vi "Set__slk_mt.vi"(7 "values":string[][](array[string]), 8 "error in (no error)":errorcluster, 11 "ring in":refnum<class "Ring__slk_mt.lvclass">) -> (0 "error out":errorcluster, 3 "ring out":refnum<class "Ring__slk_mt.lvclass">)   [LabVIEW 2013, in "Lazyboots Menu Tool.lvlib" / "Ring__slk_mt.lvclass"]
doc: "Sets the values to the control on GUI.\n\n<b>Values:</b>\n[ [Section, Key, Value], [Section, Key, Value], ..., [Section, Key, Value] ]"
uses:
  Ring__slk_mt.lvclass
  TypeDef/TypeDef_ConnectorPattern__slk_mt.ctl
  Library/Lazyboots Menu Tool.lvlib
panel:
  # "Set__slk_mt.vi\nSets the values to the control on GUI.\n\nNOTICE -- YOU MUST LEAVE THIS NOTICE IN PLACE.\n\nCopyright (c) 2011, LIANG LIU Shawn.Liu.cn@gmail.com\nAll rights reserved.\n\nRedistribution and use in source and binary forms, with or without modification, are permitted provided that the following conditions are met:\n-Redistributions of source code must retain the above copyright notice, this list of conditions and the following disclaimer.\n-Redistributions in binary form must reproduce the above copyright notice, this list of conditions and the following disclaimer in the documentation and/or other materials provided with the distribution.\n-Neither the name of the eLp nor the names of its contributors may be used to endorse or promote products derived from this software without specific prior written permission.\n\nTHIS SOFTWARE IS PROVIDED BY THE COPYRIGHT HOLDERS AND CONTRIBUTORS \"AS IS\" AND ANY EXPRESS OR IMPLIED WARRANTIES, INCLUDING, BUT NOT LIMITED TO, THE IMPLIED WARRANTIES OF MERCHANTABILITY AND FITNESS FOR A PARTICULAR PURPOSE ARE DISCLAIMED. IN NO EVENT SHALL THE COPYRIGHT HOLDER OR CONTRIBUTORS BE LIABLE FOR ANY DIRECT, INDIRECT, INCIDENTAL, SPECIAL, EXEMPLARY, OR CONSEQUENTIAL DAMAGES (INCLUDING, BUT NOT LIMITED TO, PROCUREMENT OF SUBSTITUTE GOODS OR SERVICES; LOSS OF USE, DATA, OR PROFITS; OR BUSINESS INTERRUPTION) HOWEVER CAUSED AND ON ANY THEORY OF LIABILITY, WHETHER IN CONTRACT, STRICT LIABILITY, OR TORT (INCLUDING NEGLIGENCE OR OTHERWISE) ARISING IN ANY WAY OUT OF THE USE OF THIS SOFTWARE, EVEN IF ADVISED OF THE POSSIBILITY OF SUCH DAMAGE."
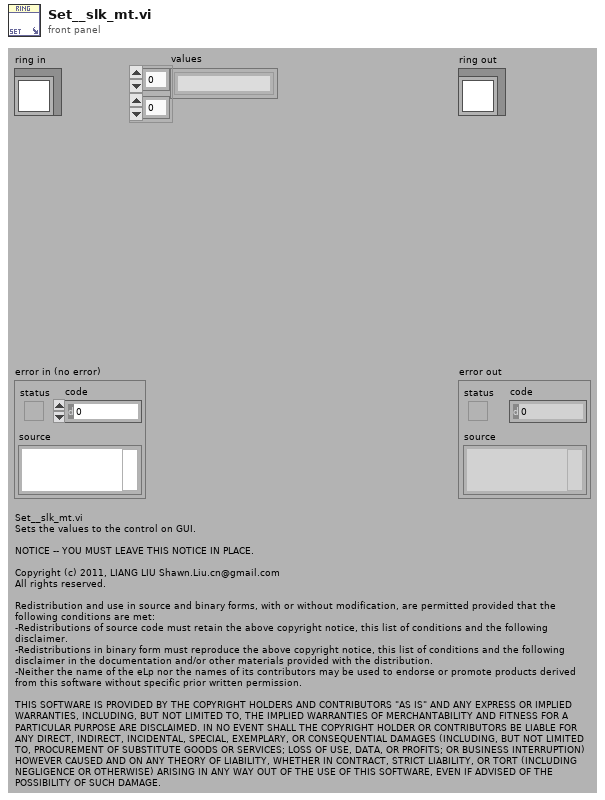
[diagram p1: front panel]
types:
  T1 = typedef "Lazyboots Menu Tool.lvlib/TypeDef_ConnectorPattern__slk_mt.ctl" = u16
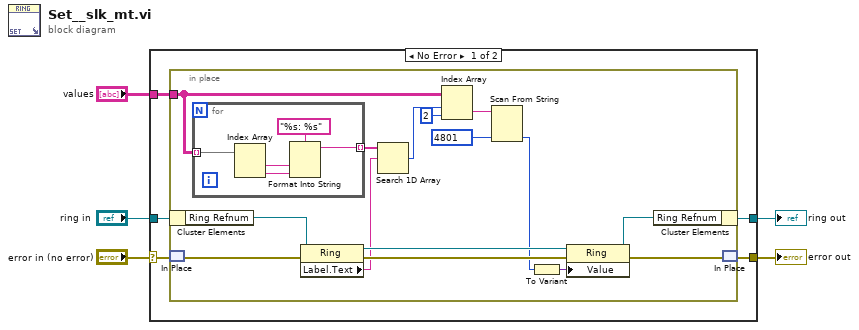
[diagram p0: block diagram]
diagram:
  n1 = case shown="No Error" "error in (no error)" {
    selector: "error in (no error)" -> [w7 w32]
    tunnel: "values" -> [w10 _]
    tunnel: "ring in" -> [w9 w31]
    tunnel: [w8 w32] -> w3
    tunnel: [w6 w31] -> w1
    frame No Error {
      n2 = in-place {
        in-place-border: w10 -> [w19]
        w17 = T1 4801 items=["4801"=4801, "4805"=4805, "4810"=4810, "4812"=4812, "4815"=4815, "4820"=4820, "4826"=4826, "4833"=4833, "4834"=4834, "4835"=4835] ("Add Error: Connector Pattern")
        n3 = in-place-cluster #1(w9) -> ("Ring Refnum"=w14:refnum<vi>)
        n4 = in-place-match #2(w7) -> (w11:errorcluster)
        n5 = for {
          tunnel: w19 -> [w30] mode=indexing
          tunnel: [w26] -> w25 mode=indexing
          n6 = Index Array(array=w30) -> (element #1=w28:string, element #2=w27:string)  [unwired: 2 in]
          n7 = Format Into String(format string="%s: %s", w28, w27) -> (resulting string=w26:string)  [unwired: 2 in, 1 out]
        }
        n8 = property class="Ring"(reference=w14, error in=w11) -> (reference out=w21:refnum<vi>, error out=w22:errorcluster, "Label.Text"=w20:string)
        n9 = Search 1D Array(1D array=w25, element=w20) -> (index of element=w23:i32)  [unwired: 1 in]
        n10 = Index Array(array=w19, index (row)=w23, index (col)=2 ("disabled index (col)")) -> (element=w18:string)
        n11 = Scan From String(input string=w18, default 1=w17) -> (output 1=w16:T1)  [unwired: 3 in, 3 out]
        n12 = To Variant(anything=w16) -> (Variant=w15:variant)
        n13 = property class="Ring"(reference=w21, error in=w22, "Value"=w15) -> (reference out=w13:refnum<vi>, error out=w12:errorcluster)
        n14 = in-place-cluster #1("Ring Refnum"=w13) -> (w6:refnum<class "Ring__slk_mt.lvclass">)
        n15 = in-place-match #2(w12) -> (w8:errorcluster)
      }
    }
    frame Error {
    }
  }
  "error out" <- w3
  "ring out" <- w1
